vi "Lex Text.vi"(8 "Error In":errorcluster) -> (0 "Error Out":errorcluster)   [LabVIEW 2018, in "Tests.lvlib" / "Lexer.lvlib"]
uses:
  Lexer.lvlib
  src/Toolkit/Low-Level/Tokens/Text/Text.lvclass
  src/Toolkit/Low-Level/Support/Lex String.vi
  <vilib>/Utility/LVClass/Get LV Class Name.vi
  src/Toolkit/Low-Level/Tokens/Contentable/Contentable.lvclass
  <vilib>/addons/_JKI Toolkits/Caraya/classes/Test/Test.lvclass
  <vilib>/addons/_JKI Toolkits/Caraya/classes/Assert/Assert.lvclass
  Tests.lvlib
  src/Toolkit/Toolkit.lvlib
  src/Toolkit/Low-Level/Tokens/Token/Token.lvclass
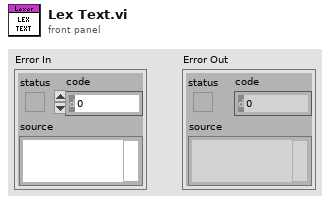
[diagram p1: front panel]
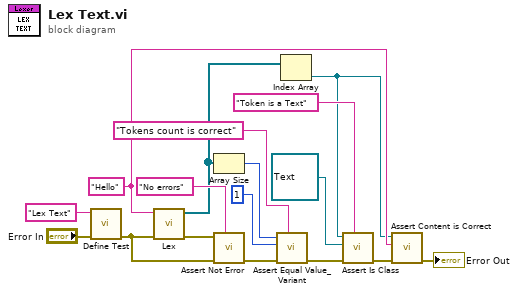
[diagram p0: block diagram]
diagram:
  w5 = "Hello" ("String")
  n1 = call <vilib>:"Define Test.vi"("error in (no error)"="Error In", "Label (VI Title)"="Lex Text") -> ("error out"=w2:errorcluster)  [unwired: 9 in]
  n2 = call-poly "Lex.vi"("Error In"=w2, "Input"=w5) -> ("Error Out"=w15:errorcluster, "Tokens"=w1:refnum<class "Token.lvclass">[])  [unwired: 8 in]
  n3 = Array Size(array=w1) -> (size(s)=w11:i32)
  n4 = call <vilib>:"Assert Not Error.vi"("Label"="No errors", "error in (no error)"=w2, "Not Error?"=w15) -> ("error out"=w13:errorcluster)  [unwired: 8 in]
  n5 = call <vilib>:"Assert Equal Value_Variant.vi"("Label"="Tokens count is correct", "error in (no error)"=w13, "Y"=1 ("size(s)"), "X"=w11) -> ("error out"=w9:errorcluster)  [unwired: 7 in]
  n6 = Index Array(array=w1) -> (element=w3:refnum<class "Token.lvclass">)  [unwired: 1 in]
  n7 = call "Assert Is Class.vi"("Label"="Token is a Text", "Error In"=w9, "Expected"=refnum<class "Text.lvclass"> refnum ("Mustache.lvlib:Tokens.lvlib:Text.lvclass"), "Actual"=w3) -> ("Error Out"=w4:errorcluster)  [unwired: 7 in]
  n8 = call "Assert Content is Correct.vi"("Error In"=w4, "Expected"=w5, "Token"=w3) -> ("Error Out"=→"Error Out":errorcluster)  [unwired: 8 in]
